vi "Summation of N Numbers.vi"() -> ()   [LabVIEW 2014]
panel:
  out "Count":i32
  out "Sum":i32
  in  "N":u8=10
  # "Summation of N Numbers"
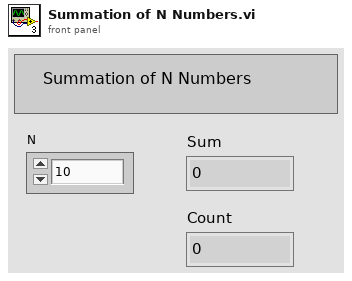
[diagram p1: front panel]
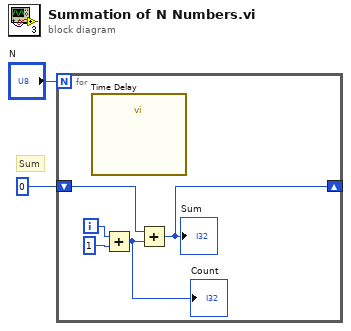
[diagram p0: block diagram]
diagram:
  # "Sum"
  n1 = for {
    N: "N" -> [_]
    shift-right: [w5] -> _
    shift-left: 0 -> [w6]
    i -> [w4]
    n2 = call "Time Delay"() -> ()  [unwired: 11 in, 1 out]
    n3 = Add(x=w4, y=1) -> (x+y=w3:i32)
    "Count" <- w3
    n4 = Add(x=w6, y=w3) -> (x+y=w5:i32)
    "Sum" <- w5
  }
